vi "Init.vi"(8 "error in":errorcluster, 10 "Variant":variant, 11 "Editor Base in":refnum<class "Editor Control Base.lvclass">) -> (0 "error out":errorcluster, 3 "Editor Base out":refnum<class "Editor Control Base.lvclass">)   [LabVIEW 2024, in "SourceGrid.lvlib" / "Editor Control Base.lvclass"]
uses:
  Editor Control Base.lvclass
  Editor Control Base.lvclass/Editor Control Base.ctl
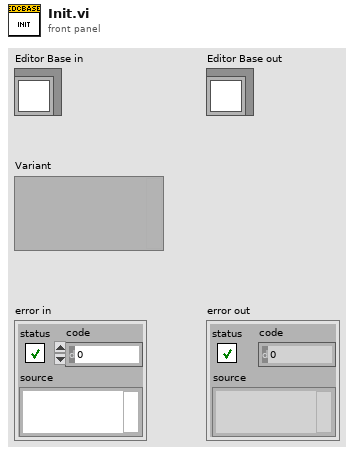
[diagram p1: front panel]
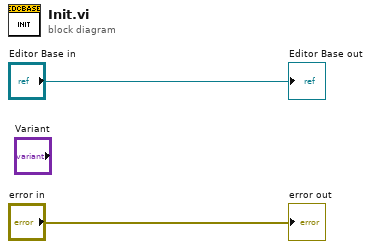
[diagram p0: block diagram]
diagram:
  "error out" <- "error in"
  "Editor Base out" <- "Editor Base in"
